vi "angle to pulse.vi"(11 "Angle":dbl) -> (1 "lo(x)":u16, 2 "hi(x)":u16, 3 "Pulses":u32)   [LabVIEW 2025, in "Motor.lvlib" / "CL57RS.lvclass"]
uses:
  CL57RS.lvclass
  CL57RS.lvclass/CL57RS.ctl
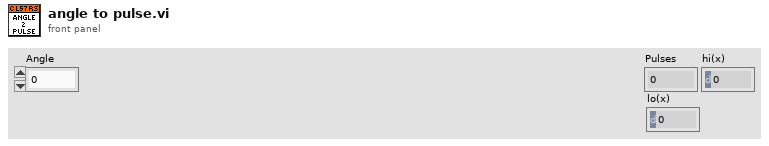
[diagram p1: front panel]
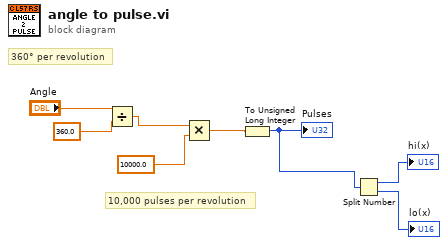
[diagram p0: block diagram]
diagram:
  # "360° per revolution"
  # "10,000 pulses per revolution"
  n1 = Divide(x="Angle", y=360.0) -> (x/y=w6:dbl)
  n2 = Multiply(x=w6, y=10000.0) -> (x*y=w4:dbl)
  n3 = To Unsigned Long Integer(number=w4) -> (unsigned 32bit integer=w3:u32)
  "Pulses" <- w3
  n4 = Split Number(x=w3) -> (hi(x)=→"hi(x)":u16, lo(x)=→"lo(x)":u16)
